vi "Read MissionOp Index Msg.vi"(8 "error in (no error)":errorcluster, 11 "Mission Set Op Index and Run Msg in":refnum<class "Mission Set Op Index and Run Msg.lvclass">) -> (0 "error out":errorcluster, 2 "MissionOp Index":i32, 3 "Mission Set Op Index and Run Msg out":refnum<class "Mission Set Op Index and Run Msg.lvclass">)   [LabVIEW 2015, in "RDS Child Messages.lvlib" / "Mission Set Op Index and Run Msg.lvclass"]
uses:
  Mission Set Op Index and Run Msg.lvclass
  Mission Set Op Index and Run Msg.lvclass/Mission Set Op Index and Run Msg.ctl
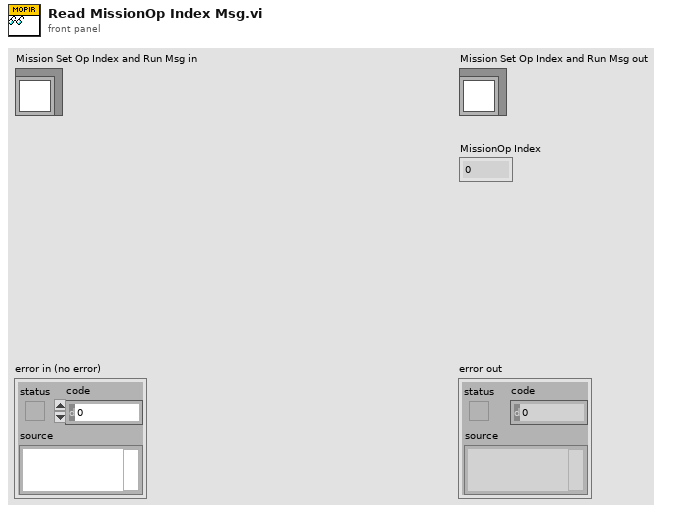
[diagram p1: front panel]
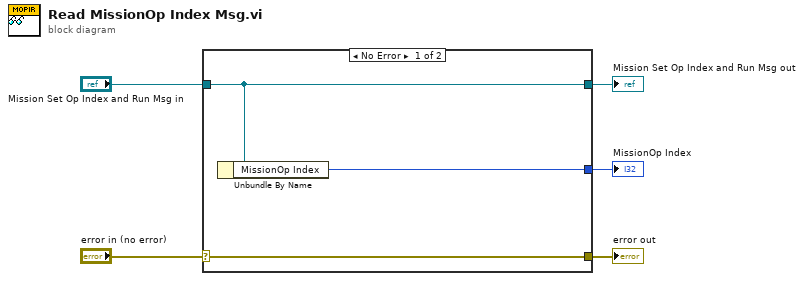
[diagram p0: block diagram]
diagram:
  n1 = case shown="No Error" "error in (no error)" {
    selector: "error in (no error)" -> [w8 w9]
    tunnel: [w8 w9] -> w4
    tunnel: [w7 w10] -> w2
    tunnel: "Mission Set Op Index and Run Msg in" -> [w7 w10]
    tunnel: [w6 _] -> w1
    frame No Error {
      n2 = Unbundle By Name(w7) -> ("MissionOp Index"=w6:i32)
    }
    frame Error {
    }
  }
  "error out" <- w4
  "Mission Set Op Index and Run Msg out" <- w2
  "MissionOp Index" <- w1
